vi "Avery Weight Tronix Modbus 32bit Number Combine.vi"(11 "Holding Registers":u16[](array[numeric])) -> (2 "word swapped":u32, 3 "Modbus Float":sgl)   [LabVIEW 2016]
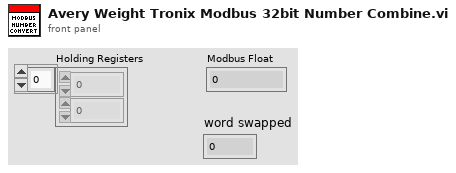
[diagram p1: front panel]
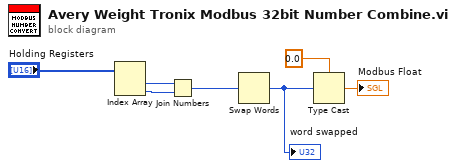
[diagram p0: block diagram]
diagram:
  n1 = Index Array(array="Holding Registers") -> (element #1=w1:u16, element #2=w5:u16)  [unwired: 2 in]
  n2 = Join Numbers(hi=w1, lo=w5) -> ((hi.lo)=w2:u32)
  n3 = Swap Words(1:w2) -> (0:w3:u32)
  "word swapped" <- w3
  n4 = Type Cast(type=sgl 0.0, x=w3) -> (*(type *) &x=→"Modbus Float":sgl)
